vi "Interpret DataType.vi"(11 "NI_DataType":u32) -> (3 "TDMS Data Type":T1)   [LabVIEW 2020, in "TDMS.lvlib"]
doc: "Translate the NI_DataType to a TDMS Data Type enum."
uses:
  TDMS.lvlib
  Controls/Ctl_DataType.ctl
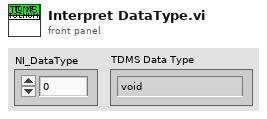
[diagram p1: front panel]
types:
  T1 = typedef "TDMS.lvlib/Ctl_DataType.ctl" = enum16{"void", "int8", "int16", "int32", "int64", "uint8", "uint16", "uint32", "uint64", "single", "double", "extended float", "single with unit", "double with unit", "extended float with unit", "string", "logical", "timestamp", "DAQmx"}
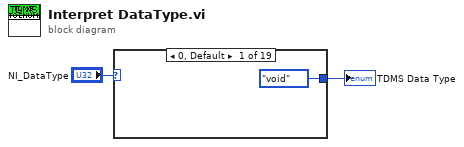
[diagram p0: block diagram]
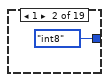
[diagram p2: hidden frame]
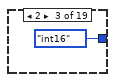
[diagram p3: hidden frame]
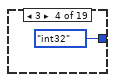
[diagram p4: hidden frame]
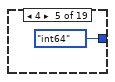
[diagram p5: hidden frame]
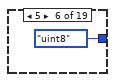
[diagram p6: hidden frame]
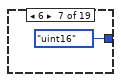
[diagram p7: hidden frame]
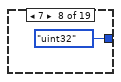
[diagram p8: hidden frame]
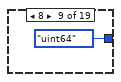
[diagram p9: hidden frame]
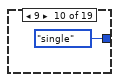
[diagram p10: hidden frame]
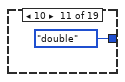
[diagram p11: hidden frame]
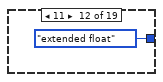
[diagram p12: hidden frame]
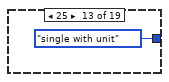
[diagram p13: hidden frame]
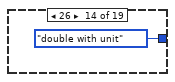
[diagram p14: hidden frame]
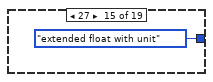
[diagram p15: hidden frame]
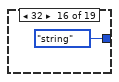
[diagram p16: hidden frame]
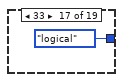
[diagram p17: hidden frame]
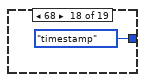
[diagram p18: hidden frame]
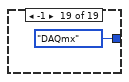
[diagram p19: hidden frame]
diagram:
  n1 = case shown="0, Default" "NI_DataType" {
    tunnel: [Ctl_DataType."void" ("TDMS Data Type") Ctl_DataType."int8" ("TDMS Data Type") Ctl_DataType."int16" ("TDMS Data Type") Ctl_DataType."int32" ("TDMS Data Type") Ctl_DataType."int64" ("TDMS Data Type") Ctl_DataType."uint8" ("TDMS Data Type") Ctl_DataType."uint16" ("TDMS Data Type") Ctl_DataType."uint32" ("TDMS Data Type") Ctl_DataType."uint64" ("TDMS Data Type") Ctl_DataType."single" ("TDMS Data Type") Ctl_DataType."double" ("TDMS Data Type") Ctl_DataType."extended float" ("TDMS Data Type") Ctl_DataType."single with unit" ("TDMS Data Type") Ctl_DataType."double with unit" ("TDMS Data Type") Ctl_DataType."extended float with unit" ("TDMS Data Type") Ctl_DataType."string" ("TDMS Data Type") Ctl_DataType."logical" ("TDMS Data Type") Ctl_DataType."timestamp" ("TDMS Data Type") Ctl_DataType."DAQmx" ("TDMS Data Type")] -> w1
    frame 0, Default {
    }
    frame 1 {
    }
    frame 2 {
    }
    frame 3 {
    }
    frame 4 {
    }
    frame 5 {
    }
    frame 6 {
    }
    frame 7 {
    }
    frame 8 {
    }
    frame 9 {
    }
    frame 10 {
    }
    frame 11 {
    }
    frame 25 {
    }
    frame 26 {
    }
    frame 27 {
    }
    frame 32 {
    }
    frame 33 {
    }
    frame 68 {
    }
    frame -1 {
    }
  }
  "TDMS Data Type" <- w1
